vi "Popup.vi"(8 "error in (no error)":errorcluster, 9 "Panel":refnum<class "Panel.lvclass">, 10 "String in":string, 11 "No Popup Data Type in":refnum<class "No Popup Data Type.lvclass">) -> (0 "error out":errorcluster, 2 "String out":string, 3 "No Popup Data Type out":refnum<class "No Popup Data Type.lvclass">)   [LabVIEW 2018, in "No Popup Data Type.lvclass"]
uses:
  No Popup Data Type.lvclass
  <vilib>/MGI/Panel Manager/Panel/Panel/Panel.lvclass
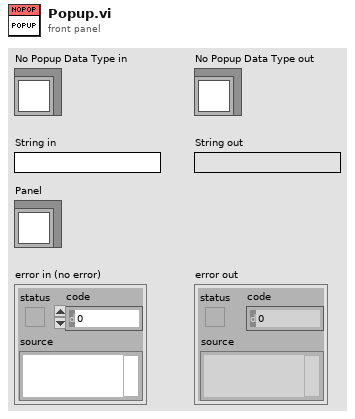
[diagram p1: front panel]
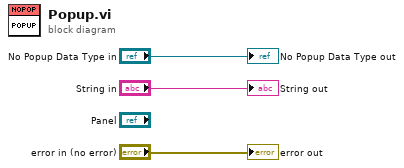
[diagram p0: block diagram]
diagram:
  "error out" <- "error in (no error)"
  "No Popup Data Type out" <- "No Popup Data Type in"
  "String out" <- "String in"
